vi "squareOrIntersection.vi"(6 "Parâmetros Ini":T3={"Gyro Port"=0, "Sensor - Left"=3, "Sensor - Right"=2, "     Color \nSensor Port"=1, "Kp Front"=0.5, "Motor speed"=-15, "Distance to street"=0.0, "Motor speed turns"=16, "Kp Curvas"=0.0} {"Kp Front" format="%.3f"; "Color \nSensor Port" items=["Port 1", "Port 2", "Port 3", "Port 4"]; "Sensor - Right" items=["Port 1", "Port 2", "Port 3", "Port 4"]; "Sensor - Left" items=["Port 1", "Port 2", "Port 3", "Port 4"]; "Gyro Port" items=["Port 1", "Port 2", "Port 3", "Port 4"]}, 10 "NXT/EV3":T2) -> (1 "CS":enum16{"Street", "Intersection", "End", "Stop"}(ring))   [LabVIEW 2016]
uses:
  <vilib>/NXT/Subs/LVHSConnector.ctl
  <vilib>/NXT/LegoClasses/BrickReference/BrickReference.lvclass
  <vilib>/NXT/Subs/ColorSensorColors.ctl
  parametros.ctl
  <vilib>/NXT/Block Support/NXT_InputPort.ctl
  <vilib>/NXT/Block Support/NXT_OutputPort.ctl
  <vilib>/NXT/NXTIO Xnodes/NXTIONodeSubVIs/NXTMoveMotors.vi
  <vilib>/NXT/NXTIO Xnodes/NXTIONodeSubVIs/NXTStopMotors.vi
  <vilib>/NXT/NXTIO Xnodes/AddressXNode/NXTIOAddress.xnode
  <vilib>/NXT/NXTIO Xnodes/NXTIOXNode/NXTIO.xnode
panel:
  in  "Contador de cores 1":dbl
  out "Numeric":i32
  out "Array":T1[](array[typedef])
  out "NXT/EV3 2":T2
  out "Detected Color":T1
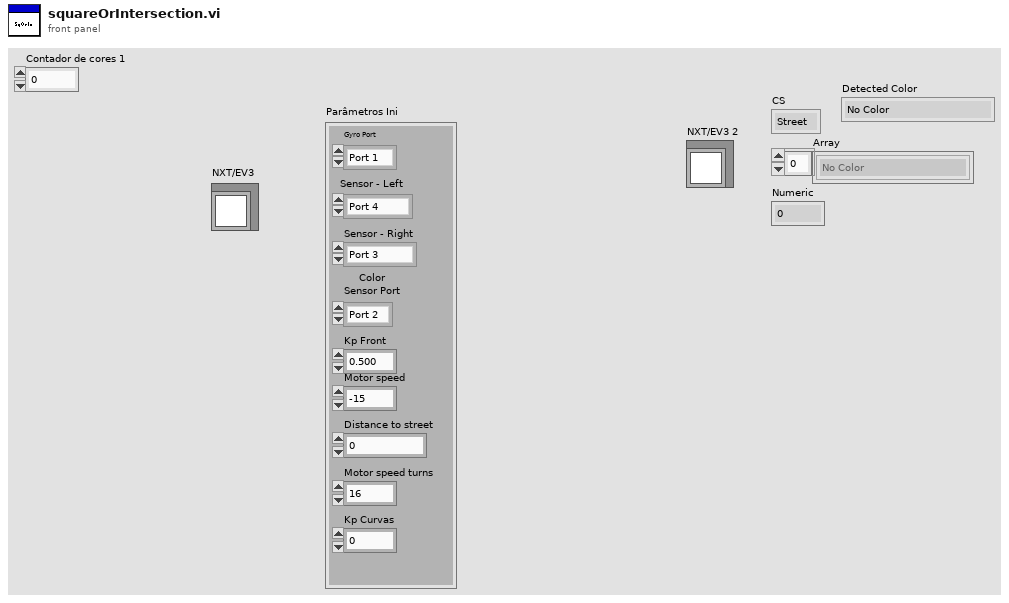
[diagram p1: front panel]
types:
  T1 = typedef "ColorSensorColors.ctl" = enum16{"No Color", "Black", "Blue", "Green", "Yellow", "Red", "White", "Brown"}
  T2 = typedef "LVHSConnector.ctl" = refnum<class "BrickReference.lvclass">
  T3 = typedef "parametros.ctl" = cluster{"Gyro Port":T4, "Sensor - Left":T4, "Sensor - Right":T4, "     Color \nSensor Port":T4, "Kp Front":dbl, "Motor speed":i32, "Distance to street":dbl, "Motor speed turns":i32, "Kp Curvas":dbl}
  T4 = typedef "NXT_InputPort.ctl" = u32
  T5 = typedef "NXT_OutputPort.ctl" = u8
  T6 = enum16{"Street", "Intersection", "End", "Stop", "Square", "Delivery"}
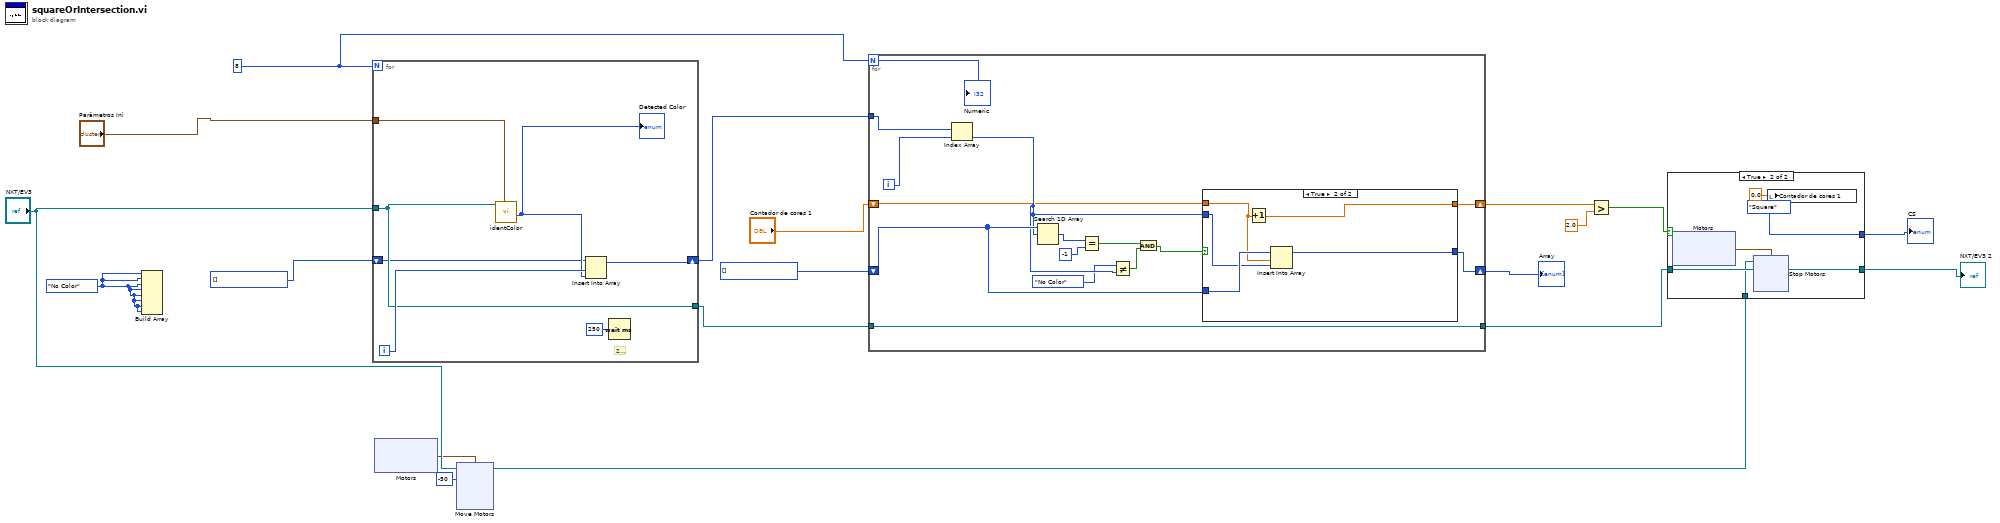
[diagram p0: block diagram]
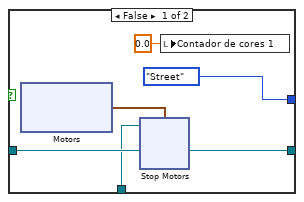
[diagram p2: hidden frame]
diagram:
  w3 = T1[] [] items=["No Color", "Black", "Blue", "Green", "Yellow", "Red", "White", "Brown"] ("array")
  w5 = T1[] [] items=["No Color", "Black", "Blue", "Green", "Yellow", "Red", "White", "Brown"] ("array")
  w6 = ColorSensorColors."No Color" ("Detected Color")
  w8 = i8 -50 ("Power/Speed 1")
  w18 = 8
  n1 = Build Array(w6, w6, w6, w6, w6, w6, w6, w6) -> ()  [unwired: 1 out]
  n2 = for {
    N: w18 -> [_]
    shift-right: [w25] -> w19
    shift-left: w5 -> [w20]
    tunnel: "Parâmetros Ini" -> [w23]
    tunnel: [w21] -> w13
    tunnel: "NXT/EV3" -> [w21]
    i -> [w26]
    # "250"
    n3 = call "identColor.vi"("Parâmetros Ini"=w23, "NXT/EV3"=w21) -> ("Collor"=w24:T1)  [unwired: 9 in]
    "Detected Color" <- w24
    n4 = Insert Into Array(array=w20, index=w26, new element=w24) -> (w25:T1[])
    n5 = Wait (ms)(milliseconds to wait=u32 250) -> ()  [unwired: 1 out]
  }
  n6 = xnode "Motors"() -> ("Motor"=w9:cluster{"Port":T5, "Port":T5})
  n7 = xnode "Move Motors"("Power/Speed 2"=w8, "Power/Speed 1"=w8, "Motors"=w9, "NXT/EV3"="NXT/EV3") -> ("NXT/EV3"=w7:T2)
  n8 = for {
    N: w18 -> [w35]
    tunnel: w19 -> [w40]
    shift-right: [w37] -> w4
    shift-left: w3 -> [w38]
    tunnel: [w36] -> w11
    tunnel: w13 -> [w36]
    shift-right: [w34] -> w2
    shift-left: "Contador de cores 1" -> [w27]
    i -> [w41]
    n9 = Index Array(array=w40, index=w41) -> (element=w30:T1)
    n10 = Search 1D Array(1D array=w38, element=w30) -> (index of element=w31:i32)  [unwired: 1 in]
    n11 = Equal?(x=w31, y=-1) -> (x = y?=w33:bool)
    n12 = Not Equal?(x=ColorSensorColors."No Color", y=w30) -> (x != y?=w32:bool)
    n13 = And(x=w33, y=w32) -> (x .and. y?=w28:bool)
    n14 = case shown="True" w28 {
      tunnel: w38 -> [w43 w48]
      tunnel: w30 -> [_ w47]
      tunnel: [w43 w46] -> w37
      tunnel: [w42 w44] -> w34
      tunnel: w27 -> [w42 w45]
      frame False {
      }
      frame True {
        n15 = Increment(x=w45) -> (x+1=w44:dbl)
        n16 = Insert Into Array(array=w48, index=w45, new element=w47) -> (w46:T1[])
      }
    }
    "Numeric" <- w35
  }
  "Array" <- w4
  n17 = Greater?(x=w2, y=2.0) -> (0:w15:bool)
  n18 = case shown="True" w15 {
    tunnel: [T6."Street" ("CS") T6."Square" ("CS")] -> w14
    tunnel: [w52 w63] -> w12
    tunnel: w11 -> [w52 w63]
    tunnel: w7 -> [w50 w61]
    frame False {
      n19 = xnode "Motors"() -> ("Motor"=w51:cluster{"Port":T5, "Port":T5})
      n20 = xnode "Stop Motors"("Motors"=w51, "NXT/EV3"=w50) -> ()  [unwired: 1 out]
      n21 = local write "Contador de cores 1"(0.0 ("Contador de cores 1")) -> ()
    }
    frame True {
      n22 = xnode "Motors"() -> ("Motor"=w62:cluster{"Port":T5, "Port":T5})
      n23 = xnode "Stop Motors"("Motors"=w62, "NXT/EV3"=w61) -> ()  [unwired: 1 out]
      n24 = local write "Contador de cores 1"(0.0 ("Contador de cores 1")) -> ()
    }
  }
  "NXT/EV3 2" <- w12
  "CS" <- w14
